vi "test_PhotonPoseEstimator_AvgBestPose.vi"(8 "error in (no error)":errorcluster) -> (0 "error out":errorcluster, 3 "Test Passed":bool)   [LabVIEW 2019]
uses:
  <vilib>/Rock Robotics/WPI/ThirdParty/JAS_Junk/TrajLib/Trajectory_Library.lvlib
  <vilib>/Rock Robotics/WPI/ThirdParty/PhotonVisionLib/PhotonVisionLib.lvlib
  <vilib>/Rock Robotics/WPI/ThirdParty/PhotonVisionLib/Enum/PhotonPoseStrategy_ENUM.ctl
  <vilib>/Rock Robotics/WPI/ThirdParty/JAS_Junk/TrajLib/TypeDef/TRANSLATION3D.ctl
  <vilib>/Rock Robotics/WPI/ThirdParty/JAS_Junk/TrajLib/TypeDef/QUATERNION.ctl
  <vilib>/Rock Robotics/WPI/ThirdParty/JAS_Junk/TrajLib/TypeDef/ROTATION3D.ctl
  <vilib>/Rock Robotics/WPI/ThirdParty/JAS_Junk/TrajLib/TypeDef/POSE3D.ctl
  <vilib>/Rock Robotics/WPI/ThirdParty/PhotonVisionLib/TypeDef/PhotonEstimatedRobotPoseType.ctl
  <vilib>/Rock Robotics/WPI/ThirdParty/PhotonVisionLib/TypeDef/TargetCornerType.ctl
  <vilib>/Rock Robotics/WPI/ThirdParty/JAS_Junk/TrajLib/TypeDef/TRANSFORM3D.ctl
  <vilib>/Rock Robotics/WPI/ThirdParty/PhotonVisionLib/TypeDef/PhotonTrackedTargetType.ctl
panel:
  out "Pos Found":bool
  out "PhotonEstimatedRobotPose":T1={"EstimatedPose"={"Translation3d"={"X"=0.0, "Y"=0.0, "Z"=0.0}, "Rotation3d"={"Q_quaternion"={"R"=1.0, "V"=[0.0, 0.0, 0.0]}}}, "TimeStamp_Seconds"=0.0, "targetsUsed"=[], "Strategy"=enum."LOWEST_AMBIGUITY"} {"targetsUsed"."AltCameraToTarget"."TRANSLATION3D"."Z" format="%14.3f"; "targetsUsed"."AltCameraToTarget"."TRANSLATION3D"."Y" format="%14.3f"; "targetsUsed"."AltCameraToTarget"."TRANSLATION3D"."X" format="%14.3f"; "targetsUsed"."BestCameraToTarget"."TRANSLATION3D"."Z" format="%14.3f"; "targetsUsed"."BestCameraToTarget"."TRANSLATION3D"."Y" format="%14.3f"; "targetsUsed"."BestCameraToTarget"."TRANSLATION3D"."X" format="%14.3f"; "EstimatedPose"."Translation3d"."Z" format="%14.3f"; "EstimatedPose"."Translation3d"."Y" format="%14.3f"; "EstimatedPose"."Translation3d"."X" format="%14.3f"}
  out "Test 0 Passed":bool
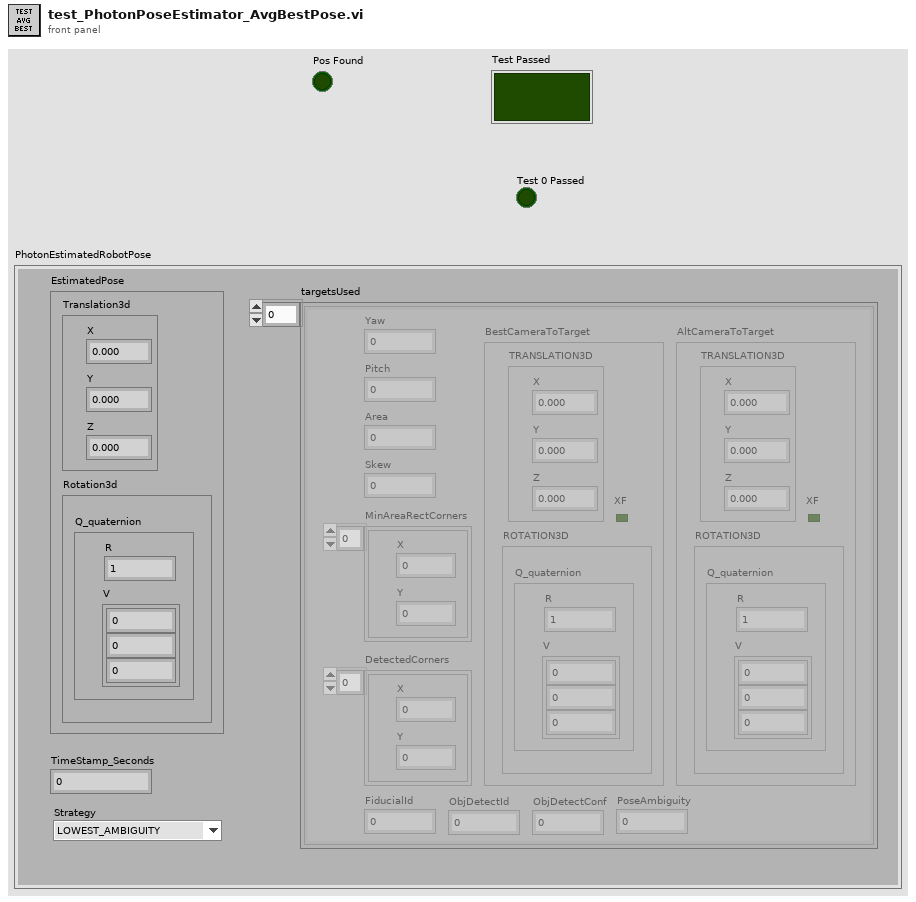
[diagram p1: front panel]
types:
  T1 = typedef "PhotonVisionLib.lvlib/PhotonEstimatedRobotPoseType.ctl" = cluster{"EstimatedPose":T2, "TimeStamp_Seconds":dbl, "targetsUsed":T6[], "Strategy":T9}
  T2 = typedef "Trajectory_Library.lvlib/POSE3D.ctl" = cluster{"Translation3d":T3, "Rotation3d":T4}
  T3 = typedef "Trajectory_Library.lvlib/TRANSLATION3D.ctl" = cluster{"X":dbl, "Y":dbl, "Z":dbl}
  T4 = typedef "Trajectory_Library.lvlib/ROTATION3D.ctl" = cluster{"Q_quaternion":T5}
  T5 = typedef "Trajectory_Library.lvlib/QUATERNION.ctl" = cluster{"R":dbl, "V":dbl[]}
  T6 = typedef "PhotonVisionLib.lvlib/PhotonTrackedTargetType.ctl" = cluster{"Yaw":dbl, "Pitch":dbl, "Area":dbl, "Skew":dbl, "MinAreaRectCorners":T7[], "BestCameraToTarget":T8, "FiducialId":i32, "AltCameraToTarget":T8, "PoseAmbiguity":dbl, "DetectedCorners":T7[], "ObjDetectId":i32, "ObjDetectConf":sgl}
  T7 = typedef "PhotonVisionLib.lvlib/TargetCornerType.ctl" = cluster{"X":dbl, "Y":dbl}
  T8 = typedef "Trajectory_Library.lvlib/TRANSFORM3D.ctl" = cluster{"TRANSLATION3D":T3, "ROTATION3D":T4, "XF":bool}
  T9 = typedef "PhotonVisionLib.lvlib/PhotonPoseStrategy_ENUM.ctl" = enum16{"LOWEST_AMBIGUITY", "CLOSEST_TO_CAMERA_HEIGHT", "CLOSEST_TO_REFERENCE_POSE", "CLOSEST_TO_LAST_POSE", "AVERAGE_BEST_TARGETS", "MULTI_TAG_PNP_ON_COPROCESSOR", "MULTI_TAG_PNP_ON_RIO"}
  T10 = typedef "Trajectory_Library.lvlib/AprilTagFieldLayout.ctl" = cluster{"AprilTagMap":map{i32, T11}, "FieldLength":dbl, "FieldWidth":dbl, "OriginPosition ":T12, "OriginPose3d":T2}
  T11 = typedef "Trajectory_Library.lvlib/AprilTag.ctl" = cluster{"ID":i32, "POSE3D":T2}
  T12 = typedef "Trajectory_Library.lvlib/AprilTagFieldLayoutOrignPosition_ENUM.ctl" = enum16{"kBlueAllianceWallRightSide,", "kRedAllianceWallRightSide,"}
  T13 = typedef "PhotonVisionLib.lvlib/PhotonPipelineMetadataType.ctl" = cluster{"CaptureTimestampMicros":i64, "PublishTimestampMicros":i64, "SequenceID":i64, "TimeSinceLastPong":i64}
  T14 = typedef "PhotonVisionLib.lvlib/PhotonPipelineResultType.ctl" = cluster{"Targets":T6[], "PhotonMultiTargetPNPResult":T15, "PhotonPipelineMetadata":T13}
  T15 = typedef "PhotonVisionLib.lvlib/PhotonMultiTargetPNPResultType.ctl" = cluster{"PhotonPNPResult":T16, "FiducialIDsUsed":i16[]}
  T16 = typedef "PhotonVisionLib.lvlib/PhotonPNPResultType.ctl" = cluster{"IsPresent":bool, "bestReprojErr":dbl, "altReprojErr":dbl, "ambiguity":dbl, "Best":T8, "Alt":T8}
  T17 = typedef "PhotonVisionLib.lvlib/PhotonPoseEstimatorType.ctl" = cluster{"LastPose":T2, "ReferencePose":T2, "FieldTags":T10, "PrimaryStratety":T9, "Camera":string, "RobotToCamera":T8, "ReportedErrors":dbl[], "HighestAmbiguity":dbl, "MultiTagFallbackStrategy":T9, "PoseCacheTimeoutSec":dbl, "PhotonTargetModel":T18, "BaseNTName":string}
  T18 = typedef "PhotonVisionLib.lvlib/PhotonTargetModel.ctl" = cluster{"Vertices":T3[], "IsPlaner":bool, "IsSpherical":bool}
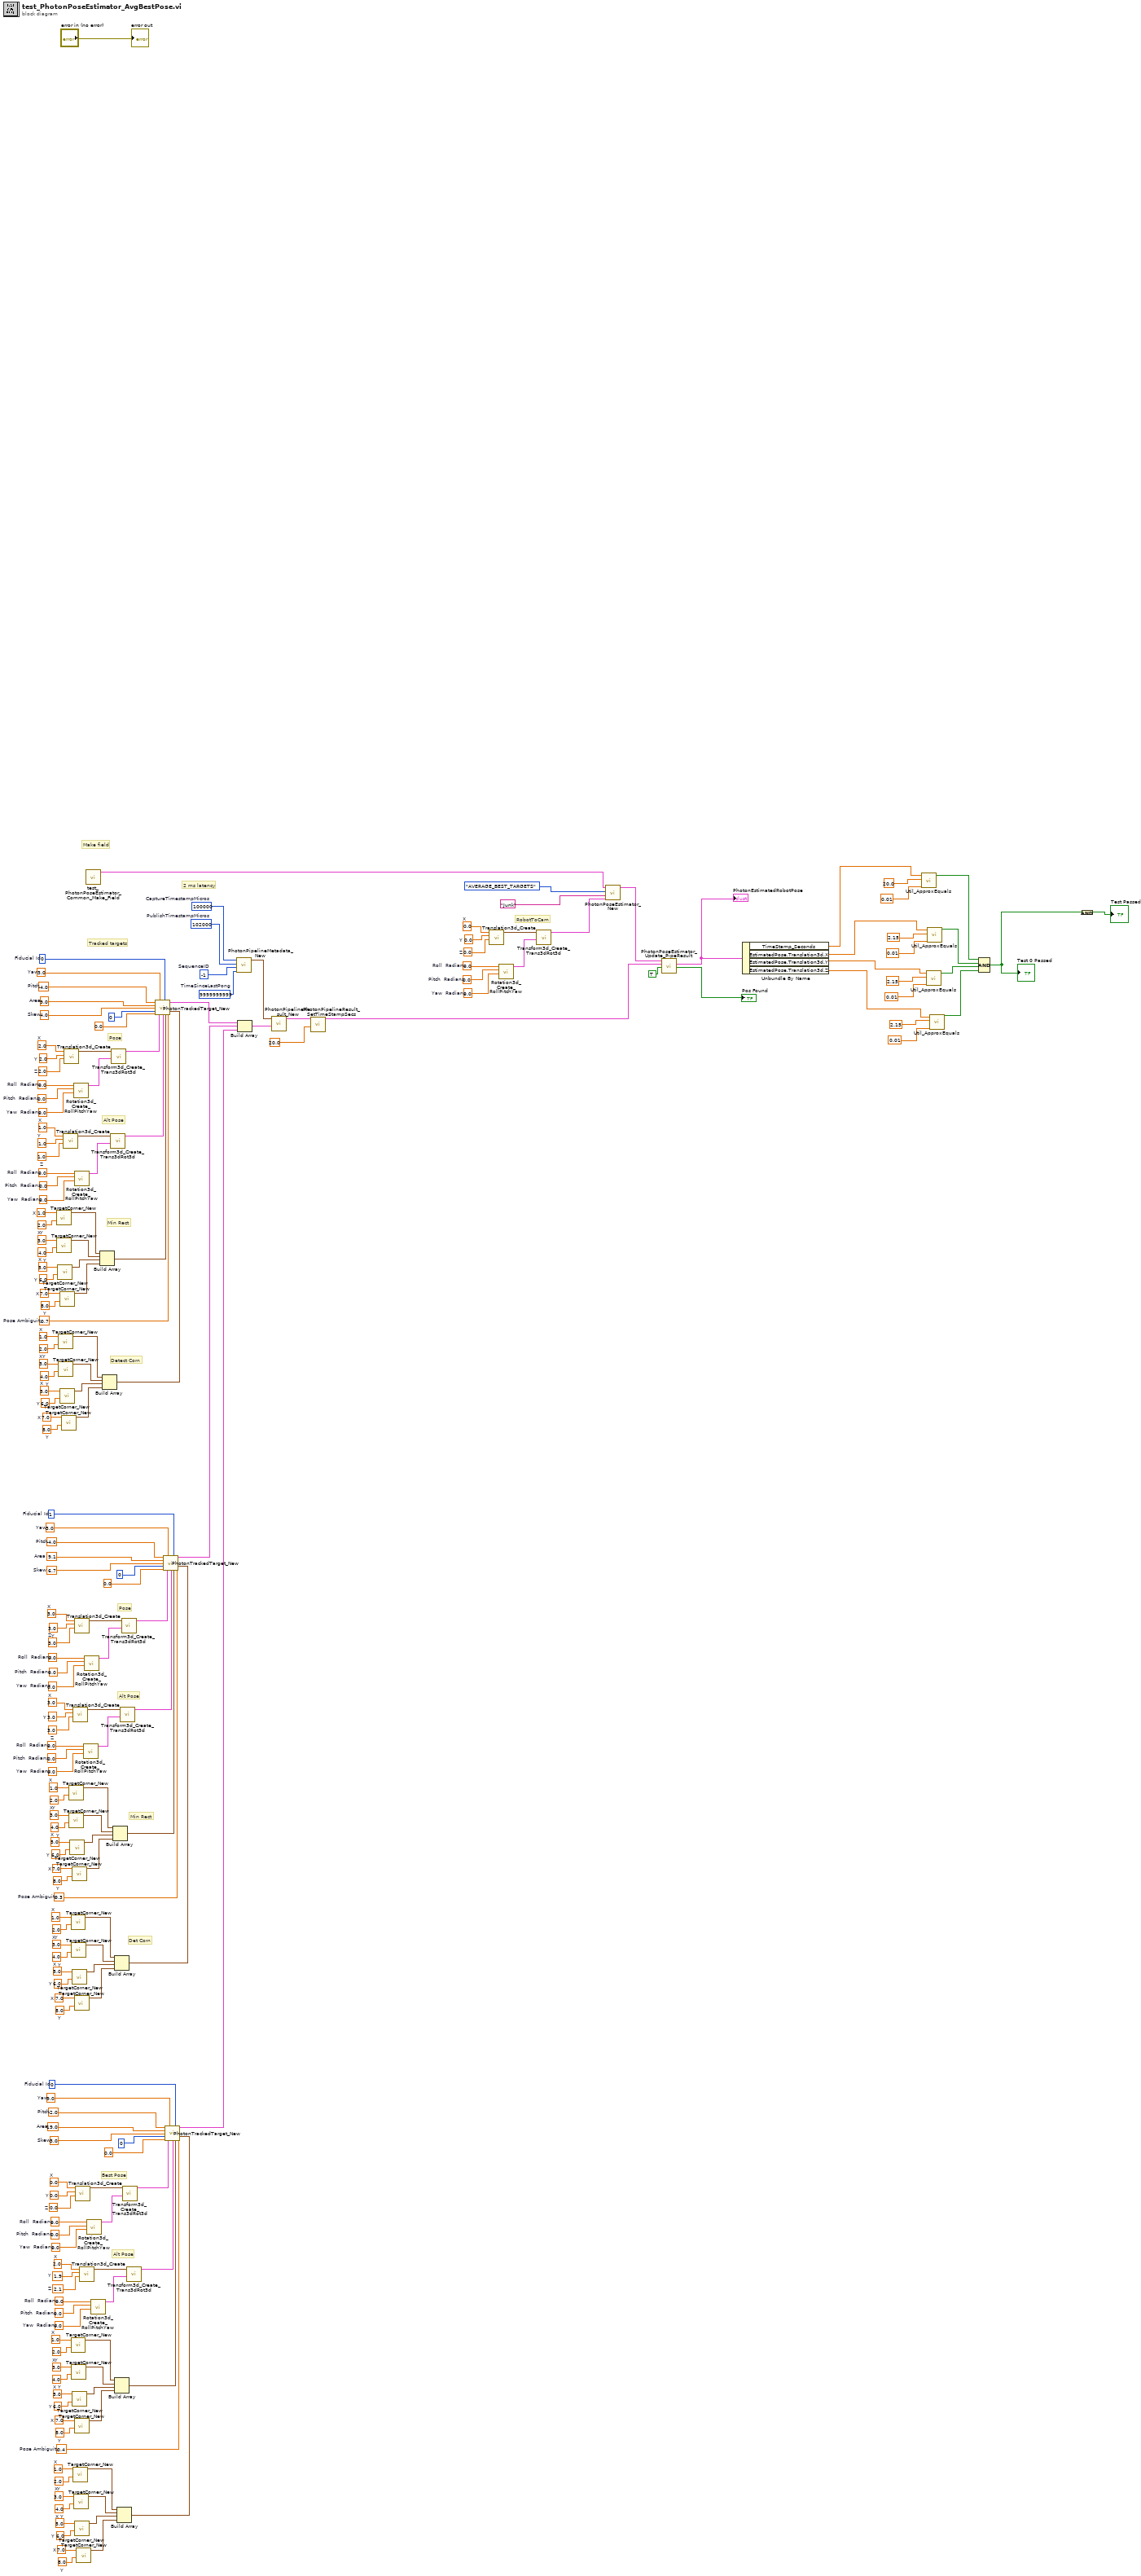
[diagram p0: block diagram]
diagram:
  w10 = i64 100000  # CaptureTimestampMicros
  w11 = i64 102000  # PublishTimestampMicros
  w12 = i64 -1  # SequenceID
  w13 = i64 9999999999  # TimeSinceLastPong
  w28 = 0.0  # Roll  Radians
  w27 = 0.0  # Pitch  Radians
  w26 = 0.0  # Yaw  Radians
  w31 = 0.0  # Z
  w30 = 0.0  # X
  w29 = 0.0  # Y
  w55 = 0.0  # Roll  Radians
  w54 = 0.0  # Pitch  Radians
  w53 = 0.0  # Yaw  Radians
  w58 = 0.0  # Z
  w57 = 0.0  # X
  w56 = 0.0  # Y
  w63 = 0.0  # Roll  Radians
  w62 = 0.0  # Pitch  Radians
  w61 = 0.0  # Yaw  Radians
  w66 = 2.1  # Z
  w65 = 2.0  # X
  w64 = 1.9  # Y
  w73 = 7.0  # X
  w74 = 8.0  # Y
  w75 = 5.0  # X
  w76 = 6.0  # Y
  w77 = 3.0  # X
  w78 = 4.0  # Y
  w79 = 1.0  # X
  w80 = 2.0  # Y
  w85 = 7.0  # X
  w86 = 8.0  # Y
  w87 = 5.0  # X
  w88 = 6.0  # Y
  w89 = 3.0  # X
  w90 = 4.0  # Y
  w91 = 1.0  # X
  w92 = 2.0  # Y
  w93 = -2.0  # Pitch
  w94 = 19.0  # Area
  w95 = 3.0  # Skew
  w96 = 0  # Fiducial Id
  w97 = 0.4  # Pose Ambiguity
  w98 = 9.0  # Yaw
  w104 = 0.0  # Roll  Radians
  w103 = 0.0  # Pitch  Radians
  w102 = 0.0  # Yaw  Radians
  w107 = 3.0  # Z
  w106 = 3.0  # X
  w105 = 3.0  # Y
  w112 = 0.0  # Roll  Radians
  w111 = 0.0  # Pitch  Radians
  w110 = 0.0  # Yaw  Radians
  w115 = 3.0  # Z
  w114 = 3.0  # X
  w113 = 3.0  # Y
  w122 = 7.0  # X
  w123 = 8.0  # Y
  w124 = 5.0  # X
  w125 = 6.0  # Y
  w126 = 3.0  # X
  w127 = 4.0  # Y
  w128 = 1.0  # X
  w129 = 2.0  # Y
  w134 = 7.0  # X
  w135 = 8.0  # Y
  w136 = 5.0  # X
  w137 = 6.0  # Y
  w138 = 3.0  # X
  w139 = 4.0  # Y
  w140 = 1.0  # X
  w141 = 2.0  # Y
  w142 = -4.0  # Pitch
  w143 = 9.1  # Area
  w144 = 6.7  # Skew
  w145 = 1  # Fiducial Id
  w146 = 0.3  # Pose Ambiguity
  w147 = 3.0  # Yaw
  w154 = 0.0  # Roll  Radians
  w153 = 0.0  # Pitch  Radians
  w152 = 0.0  # Yaw  Radians
  w157 = 2.0  # Z
  w156 = 2.0  # X
  w155 = 2.0  # Y
  w162 = 0.0  # Roll  Radians
  w161 = 0.0  # Pitch  Radians
  w160 = 0.0  # Yaw  Radians
  w165 = 1.0  # Z
  w164 = 1.0  # X
  w163 = 1.0  # Y
  w172 = 7.0  # X
  w173 = 8.0  # Y
  w174 = 5.0  # X
  w175 = 6.0  # Y
  w176 = 3.0  # X
  w177 = 4.0  # Y
  w178 = 1.0  # X
  w179 = 2.0  # Y
  w184 = 7.0  # X
  w185 = 8.0  # Y
  w186 = 5.0  # X
  w187 = 6.0  # Y
  w188 = 3.0  # X
  w189 = 4.0  # Y
  w190 = 1.0  # X
  w191 = 2.0  # Y
  w192 = -4.0  # Pitch
  w193 = 9.0  # Area
  w194 = 4.0  # Skew
  w195 = 0  # Fiducial Id
  w196 = 0.7  # Pose Ambiguity
  w197 = 3.0  # Yaw
  # "2 ms latency"
  # "RobotToCam"
  # "Det Corn"
  # "Min Rect"
  # "Pose"
  # "Detect Corn"
  # "Min Rect"
  # "Tracked targets"
  # "Make field"
  # "Best Pose"
  # "Alt Pose"
  # "Alt Pose"
  # "Pose"
  # "Alt Pose"
  n1 = call <vilib>:"TargetCorner_New.vi"("Y"=w191, "X"=w190) -> ("TargetCorner"=w183:T7)  [unwired: 9 in]
  n2 = call <vilib>:"TargetCorner_New.vi"("Y"=w189, "X"=w188) -> ("TargetCorner"=w182:T7)  [unwired: 9 in]
  n3 = call <vilib>:"TargetCorner_New.vi"("Y"=w187, "X"=w186) -> ("TargetCorner"=w181:T7)  [unwired: 9 in]
  n4 = call <vilib>:"TargetCorner_New.vi"("Y"=w179, "X"=w178) -> ("TargetCorner"=w171:T7)  [unwired: 9 in]
  n5 = call <vilib>:"TargetCorner_New.vi"("Y"=w177, "X"=w176) -> ("TargetCorner"=w170:T7)  [unwired: 9 in]
  n6 = call <vilib>:"TargetCorner_New.vi"("Y"=w185, "X"=w184) -> ("TargetCorner"=w180:T7)  [unwired: 9 in]
  n7 = call <vilib>:"TargetCorner_New.vi"("Y"=w175, "X"=w174) -> ("TargetCorner"=w169:T7)  [unwired: 9 in]
  n8 = call <vilib>:"TargetCorner_New.vi"("Y"=w173, "X"=w172) -> ("TargetCorner"=w168:T7)  [unwired: 9 in]
  n9 = call <vilib>:"Translation3d_Create.vi"("Z"=w165, "Y"=w163, "X"=w164) -> ("TRANSLATION3D"=w159:T3)  [unwired: 8 in]
  n10 = call <vilib>:"Translation3d_Create.vi"("Z"=w157, "Y"=w155, "X"=w156) -> ("TRANSLATION3D"=w151:T3)  [unwired: 8 in]
  n11 = call <vilib>:"TargetCorner_New.vi"("Y"=w141, "X"=w140) -> ("TargetCorner"=w133:T7)  [unwired: 9 in]
  n12 = call <vilib>:"TargetCorner_New.vi"("Y"=w139, "X"=w138) -> ("TargetCorner"=w132:T7)  [unwired: 9 in]
  n13 = call <vilib>:"TargetCorner_New.vi"("Y"=w137, "X"=w136) -> ("TargetCorner"=w131:T7)  [unwired: 9 in]
  n14 = call <vilib>:"TargetCorner_New.vi"("Y"=w129, "X"=w128) -> ("TargetCorner"=w121:T7)  [unwired: 9 in]
  n15 = call <vilib>:"TargetCorner_New.vi"("Y"=w92, "X"=w91) -> ("TargetCorner"=w84:T7)  [unwired: 9 in]
  n16 = call <vilib>:"TargetCorner_New.vi"("Y"=w127, "X"=w126) -> ("TargetCorner"=w120:T7)  [unwired: 9 in]
  n17 = call <vilib>:"TargetCorner_New.vi"("Y"=w90, "X"=w89) -> ("TargetCorner"=w83:T7)  [unwired: 9 in]
  n18 = call <vilib>:"TargetCorner_New.vi"("Y"=w135, "X"=w134) -> ("TargetCorner"=w130:T7)  [unwired: 9 in]
  n19 = call <vilib>:"TargetCorner_New.vi"("Y"=w125, "X"=w124) -> ("TargetCorner"=w119:T7)  [unwired: 9 in]
  n20 = call <vilib>:"TargetCorner_New.vi"("Y"=w88, "X"=w87) -> ("TargetCorner"=w82:T7)  [unwired: 9 in]
  n21 = call <vilib>:"Translation3d_Create.vi"("Z"=w115, "Y"=w113, "X"=w114) -> ("TRANSLATION3D"=w109:T3)  [unwired: 8 in]
  n22 = call <vilib>:"TargetCorner_New.vi"("Y"=w80, "X"=w79) -> ("TargetCorner"=w72:T7)  [unwired: 9 in]
  n23 = call <vilib>:"Rotation3d_Create_RollPitchYaw.vi"("Yaw"=w152, "Pitch"=w153, "Roll"=w154) -> ("Rotation3d"=w150:T4)  [unwired: 8 in]
  n24 = call <vilib>:"TargetCorner_New.vi"("Y"=w78, "X"=w77) -> ("TargetCorner"=w71:T7)  [unwired: 9 in]
  n25 = call <vilib>:"Rotation3d_Create_RollPitchYaw.vi"("Yaw"=w160, "Pitch"=w161, "Roll"=w162) -> ("Rotation3d"=w158:T4)  [unwired: 8 in]
  n26 = call <vilib>:"Translation3d_Create.vi"("Z"=w107, "Y"=w105, "X"=w106) -> ("TRANSLATION3D"=w101:T3)  [unwired: 8 in]
  n27 = call <vilib>:"TargetCorner_New.vi"("Y"=w123, "X"=w122) -> ("TargetCorner"=w118:T7)  [unwired: 9 in]
  n28 = call <vilib>:"TargetCorner_New.vi"("Y"=w86, "X"=w85) -> ("TargetCorner"=w81:T7)  [unwired: 9 in]
  n29 = call <vilib>:"TargetCorner_New.vi"("Y"=w76, "X"=w75) -> ("TargetCorner"=w70:T7)  [unwired: 9 in]
  n30 = call <vilib>:"Translation3d_Create.vi"("Z"=w58, "Y"=w56, "X"=w57) -> ("TRANSLATION3D"=w52:T3)  [unwired: 8 in]
  n31 = call <vilib>:"TargetCorner_New.vi"("Y"=w74, "X"=w73) -> ("TargetCorner"=w69:T7)  [unwired: 9 in]
  n32 = call <vilib>:"Translation3d_Create.vi"("Z"=w66, "Y"=w64, "X"=w65) -> ("TRANSLATION3D"=w60:T3)  [unwired: 8 in]
  n33 = call <vilib>:"Rotation3d_Create_RollPitchYaw.vi"("Yaw"=w110, "Pitch"=w111, "Roll"=w112) -> ("Rotation3d"=w108:T4)  [unwired: 8 in]
  n34 = call <vilib>:"Rotation3d_Create_RollPitchYaw.vi"("Yaw"=w102, "Pitch"=w103, "Roll"=w104) -> ("Rotation3d"=w100:T4)  [unwired: 8 in]
  n35 = call "test_PhotonPoseEstimator_Common_Make_Field.vi"() -> ("AprilTagFieldLayout"=w43:T10)  [unwired: 11 in]
  n36 = call <vilib>:"Rotation3d_Create_RollPitchYaw.vi"("Yaw"=w53, "Pitch"=w54, "Roll"=w55) -> ("Rotation3d"=w51:T4)  [unwired: 8 in]
  n37 = call <vilib>:"Rotation3d_Create_RollPitchYaw.vi"("Yaw"=w61, "Pitch"=w62, "Roll"=w63) -> ("Rotation3d"=w59:T4)  [unwired: 8 in]
  n38 = Build Array(w183, w182, w181, w180) -> (w167:T7[])
  n39 = Build Array(w171, w170, w169, w168) -> (w166:T7[])
  n40 = call <vilib>:"Transform3d_Create_Trans3dRot3d.vi"("Rotation3d"=w158, "Translation3d"=w159) -> ("Transform3d"=w148:T8)  [unwired: 9 in]
  n41 = call <vilib>:"Transform3d_Create_Trans3dRot3d.vi"("Rotation3d"=w150, "Translation3d"=w151) -> ("Transform3d"=w149:T8)  [unwired: 9 in]
  n42 = Build Array(w133, w132, w131, w130) -> (w117:T7[])
  n43 = Build Array(w121, w120, w119, w118) -> (w116:T7[])
  n44 = Build Array(w84, w83, w82, w81) -> (w68:T7[])
  n45 = Build Array(w72, w71, w70, w69) -> (w67:T7[])
  n46 = call <vilib>:"Transform3d_Create_Trans3dRot3d.vi"("Rotation3d"=w108, "Translation3d"=w109) -> ("Transform3d"=w99:T8)  [unwired: 9 in]
  n47 = call <vilib>:"Transform3d_Create_Trans3dRot3d.vi"("Rotation3d"=w100, "Translation3d"=w101) -> ("Transform3d"=w5:T8)  [unwired: 9 in]
  n48 = call <vilib>:"Transform3d_Create_Trans3dRot3d.vi"("Rotation3d"=w51, "Translation3d"=w52) -> ("Transform3d"=w8:T8)  [unwired: 9 in]
  n49 = call <vilib>:"Transform3d_Create_Trans3dRot3d.vi"("Rotation3d"=w59, "Translation3d"=w60) -> ("Transform3d"=w50:T8)  [unwired: 9 in]
  n50 = call <vilib>:"PhotonTrackedTarget_New.vi"("Pitch"=w192, "Yaw"=w197, "Fiducial Id"=w195, "Area"=w193, "Skew"=w194, "ObjDetectId"=0, "DetectedCorners"=w166, "DetectObjConf"=sgl 0.0, "BestCameraToTarget"=w149, "AltCameraToTarget"=w148, "MinAreaRectCorners"=w167, "Pose Ambiguity"=w196) -> ("TrackedTarget"=w49:T6)  [unwired: 3 in]
  n51 = call <vilib>:"PhotonTrackedTarget_New.vi"("Pitch"=w142, "Yaw"=w147, "Fiducial Id"=w145, "Area"=w143, "Skew"=w144, "ObjDetectId"=0, "DetectedCorners"=w116, "DetectObjConf"=sgl 0.0, "BestCameraToTarget"=w5, "AltCameraToTarget"=w99, "MinAreaRectCorners"=w117, "Pose Ambiguity"=w146) -> ("TrackedTarget"=w48:T6)  [unwired: 3 in]
  n52 = call <vilib>:"PhotonTrackedTarget_New.vi"("Pitch"=w93, "Yaw"=w98, "Fiducial Id"=w96, "Area"=w94, "Skew"=w95, "ObjDetectId"=0, "DetectedCorners"=w67, "DetectObjConf"=sgl 0.0, "BestCameraToTarget"=w8, "AltCameraToTarget"=w50, "MinAreaRectCorners"=w68, "Pose Ambiguity"=w97) -> ("TrackedTarget"=w47:T6)  [unwired: 3 in]
  n53 = call <vilib>:"PhotonPipelineMetadata_New.vi"("TimeSinceLastPong"=w13, "SequenceID"=w12, "PublishTimestampMicros"=w11, "CaptureTimestampMicros"=w10) -> ("PhotonPipelineMetadata"=w9:T13)  [unwired: 7 in]
  n54 = Build Array(w49, w48, w47) -> (w46:T6[])
  n55 = call <vilib>:"PhotonPipelineResult_New.vi"("TrackedTargets"=w46, "Metadata"=w9) -> ("PhotonPipelineResult"=w45:T14)  [unwired: 9 in]
  n56 = call <vilib>:"PhotonPipelineResult_SetTimeStampSecs.vi"("TimeStampSec"=20.0, "PhotonPipelineResult"=w45) -> ("Out PhotonPipelineResult"=w16:T14)  [unwired: 9 in]
  n57 = call <vilib>:"Translation3d_Create.vi"("Z"=w31, "Y"=w29, "X"=w30) -> ("TRANSLATION3D"=w25:T3)  [unwired: 8 in]
  n58 = call <vilib>:"Rotation3d_Create_RollPitchYaw.vi"("Yaw"=w26, "Pitch"=w27, "Roll"=w28) -> ("Rotation3d"=w24:T4)  [unwired: 8 in]
  n59 = call <vilib>:"Transform3d_Create_Trans3dRot3d.vi"("Rotation3d"=w24, "Translation3d"=w25) -> ("Transform3d"=w23:T8)  [unwired: 9 in]
  n60 = call <vilib>:"PhotonPoseEstimator_New.vi"("RobotToCamera"=w23, "Camera"="Junk", "Strategy"=PhotonPoseStrategy_ENUM."AVERAGE_BEST_TARGETS", "AprilTagFieldLayout"=w43) -> ("PhotonPoseEstimator"=w17:T17)  [unwired: 7 in]
  n61 = call <vilib>:"PhotonPoseEstimator_Update_PipeResult.vi"("Has Results"=TRUE, "PipelineResult"=w16, "PhotonPoseEstimator"=w17) -> ("Pos Found"=→"Pos Found":bool, "PhotonEstimatedRobotPose"=w15:T1)  [unwired: 6 in, 1 out]
  "PhotonEstimatedRobotPose" <- w15
  n62 = Unbundle By Name(w15) -> ("TimeStamp_Seconds"=w19:dbl, "EstimatedPose.Translation3d.X"=w34:dbl, "EstimatedPose.Translation3d.Y"=w33:dbl, "EstimatedPose.Translation3d.Z"=w32:dbl)
  n63 = call <vilib>:"Util_ApproxEquals.vi"("Tolerance"=0.01, "Value 2"=20.0, "Value 1"=w19) -> ("ApproxEquals"=w20:bool)  [unwired: 8 in]
  n64 = call <vilib>:"Util_ApproxEquals.vi"("Tolerance"=0.01, "Value 2"=2.15, "Value 1"=w33) -> ("ApproxEquals"=w36:bool)  [unwired: 8 in]
  n65 = call <vilib>:"Util_ApproxEquals.vi"("Tolerance"=0.01, "Value 2"=2.15, "Value 1"=w34) -> ("ApproxEquals"=w200:bool)  [unwired: 8 in]
  n66 = call <vilib>:"Util_ApproxEquals.vi"("Tolerance"=0.01, "Value 2"=2.15, "Value 1"=w32) -> ("ApproxEquals"=w35:bool)  [unwired: 8 in]
  n67 = Compound Arithmetic op=AND(w20, w200, w36, w35) -> (w198:bool)
  "Test 0 Passed" <- w198
  n68 = Compound Arithmetic op=AND(w198) -> (→"Test Passed":bool)
  "error out" <- "error in (no error)"
